vi "Fetch Multi Eval Meas Modulation Results.vi"(0 "VISA resource name":refnum<visa-resource-name>, 5 "Instance (1)":i32=1, 7 "Result Type (Current)":i32(ring) items=["Current"=0, "Average"=1, "Standard Deviation"=3, "Maximum"=4], 11 "error in (no error)":errorcluster) -> (4 "VISA resource name out":refnum<visa-resource-name>, 6 "Reliability":i32, 8 "Out Of Tolerance":dbl format="%^.3e", 10 "Results":dbl[](array[numeric]) format="%^.3e", 15 "error out":errorcluster)   [LabVIEW 2020, in "Rohde&Schwarz CMP LR WPAN Measurement.lvlib"]
doc: "Returns the single value results.\n\nAttribute:\n-\n\nRemote-control commands:\nFETCh:WPAN:MEAS<i>:MEValuation:MODulation[:OFFSet]:CURRent?\nFETCh:WPAN:MEAS<i>:MEValuation:MODulation[:OFFSet]:AVERage?\nFETCh:WPAN:MEAS<i>:MEValuation:MODulation[:OFFSet]:MAXimum?\nFETCh:WPAN:MEAS<i>:MEValuation:MODulation[:OFFSet]:SDEViation?"
uses:
  <instrlib>/Rohde&Schwarz CMP LR WPAN Measurement/Rohde&Schwarz CMP LR WPAN Measurement.lvlib
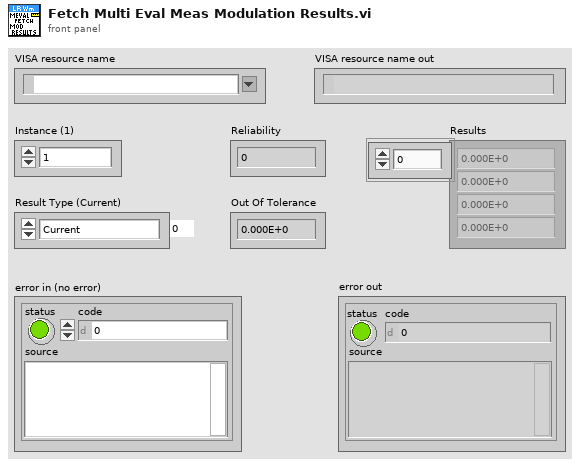
[diagram p1: front panel]
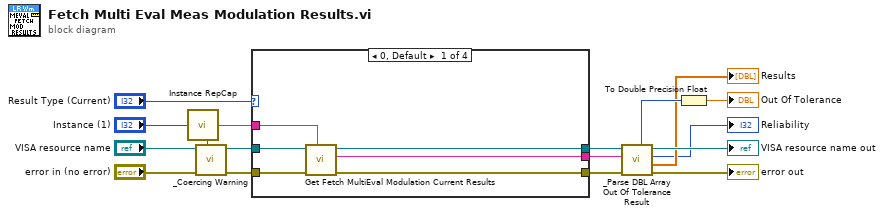
[diagram p0: block diagram]
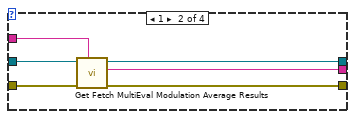
[diagram p2: hidden frame]
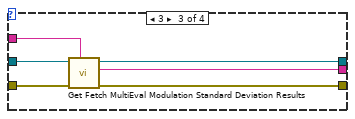
[diagram p3: hidden frame]
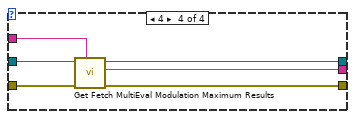
[diagram p4: hidden frame]
diagram:
  n1 = call <instrlib>:"Instance RepCap.vi"("Instance In"="Instance (1)") -> ("In Range?"=w16:bool, "RepCap Identifier Out"=w17:string)  [unwired: 1 in]
  n2 = call <instrlib>:"_Coercing Warning.vi"("In Range?"=w16, "error in (no error)"="error in (no error)", "VISA resource name"="VISA resource name") -> ("error out"=w13:errorcluster, "VISA resource name out"=w12:refnum<visa-resource-name>)  [unwired: 7 in]
  n3 = case shown="0, Default" "Result Type (Current)" {
    tunnel: w17 -> [w23 w29 w35 w41]
    tunnel: w12 -> [w22 w28 w34 w39]
    tunnel: w13 -> [w21 w27 w33 w40]
    tunnel: [w19 w25 w31 w38] -> w9
    tunnel: [w20 w26 w30 w37] -> w10
    tunnel: [w18 w24 w32 w36] -> w4
    frame 0, Default {
      n4 = call "Get Fetch MultiEval Modulation Current Results"("Repeated Capabilities"=w23, "error in (no error)"=w21, "instrument handle"=w22) -> ("error out"=w19:errorcluster, "Fetch MultiEval Modulation Current Results"=w18:string, "instrument handle out"=w20:refnum<visa-resource-name>)  [unwired: 6 in]
    }
    frame 1 {
      n5 = call "Get Fetch MultiEval Modulation Average Results"("Repeated Capabilities"=w29, "error in (no error)"=w27, "instrument handle"=w28) -> ("error out"=w25:errorcluster, "Fetch MultiEval Modulation Average Results"=w24:string, "instrument handle out"=w26:refnum<visa-resource-name>)  [unwired: 6 in]
    }
    frame 3 {
      n6 = call "Get Fetch MultiEval Modulation Standard Deviation Results"("Repeated Capabilities"=w35, "error in (no error)"=w33, "instrument handle"=w34) -> ("error out"=w31:errorcluster, "Fetch MultiEval Modulation Standard Deviation Results"=w32:string, "instrument handle out"=w30:refnum<visa-resource-name>)  [unwired: 6 in]
    }
    frame 4 {
      n7 = call "Get Fetch MultiEval Modulation Maximum Results"("Repeated Capabilities"=w41, "error in (no error)"=w40, "instrument handle"=w39) -> ("error out"=w38:errorcluster, "Fetch MultiEval Modulation Maximum Results"=w36:string, "instrument handle out"=w37:refnum<visa-resource-name>)  [unwired: 6 in]
    }
  }
  n8 = call <instrlib>:"_Parse DBL Array Out Of Tolerance Result.vi"("error in (no error)"=w9, "Input String"=w4, "VISA resource name"=w10) -> ("error out"=→"error out":errorcluster, "Results"=→"Results":dbl[], "Reliability"=→"Reliability":i32, "VISA resource name out"=→"VISA resource name out":refnum<visa-resource-name>, "Out Of Tolerance"=w7:i32)  [unwired: 4 in]
  n9 = To Double Precision Float(number=w7) -> (double precision float=→"Out Of Tolerance":dbl)
